vi "GetAppInfo.vi"(0 "App Refnum":refnum<vi>) -> (1 "VI Version":string, 2 "Application:User Name":string, 3 "Operating System:Name":string, 4 "error out":errorcluster)   [LabVIEW 2013]
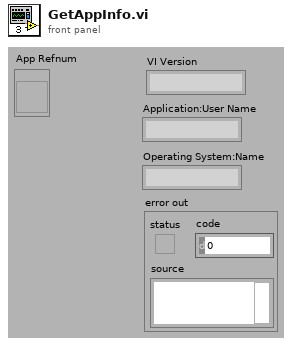
[diagram p1: front panel]
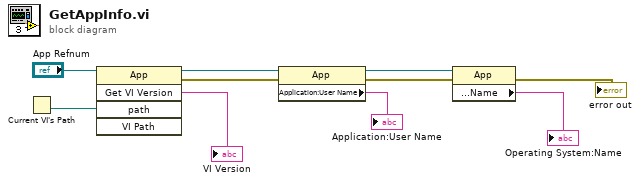
[diagram p0: block diagram]
diagram:
  n1 = Current VI's Path() -> (path=w10:path)
  n2 = invoke class="App" method="Get VI Version"(reference="App Refnum", "path"=w10) -> (reference out=w7:refnum<vi>, error out=w6:errorcluster, "GetVIVers"=→"VI Version":string)  [unwired: 3 in, 2 out]
  n3 = property class="App"(reference=w7, error in=w6) -> (reference out=w5:refnum<vi>, error out=w4:errorcluster, "Application:User Name"=→"Application:User Name":string)
  n4 = property class="App"(reference=w5, error in=w4) -> (error out=→"error out":errorcluster, "Operating System:Name"=→"Operating System:Name":string)  [unwired: 1 out]
